vi "U01_TCP_P2PWRITE.vi"() -> ()   [LabVIEW 2015]
doc: "Este VI funciona como un cliente para enviar una cadena"
panel:
  in  "Data in":string="HOLA"
  out "bytes written":i32
  out "connection ID out":refnum<k5>
  out "error out":errorcluster
  in  "IP adress":string="127.0.0.1"
  in  "Port":u16
  in  "timeout ms":i32
  in  "error in (no error)":errorcluster
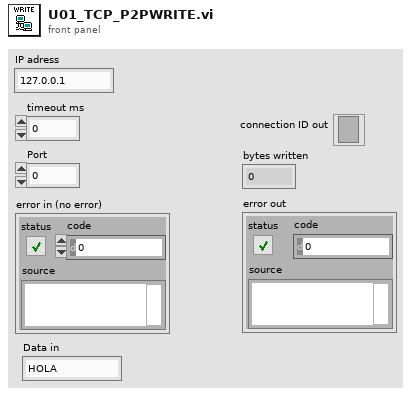
[diagram p1: front panel]
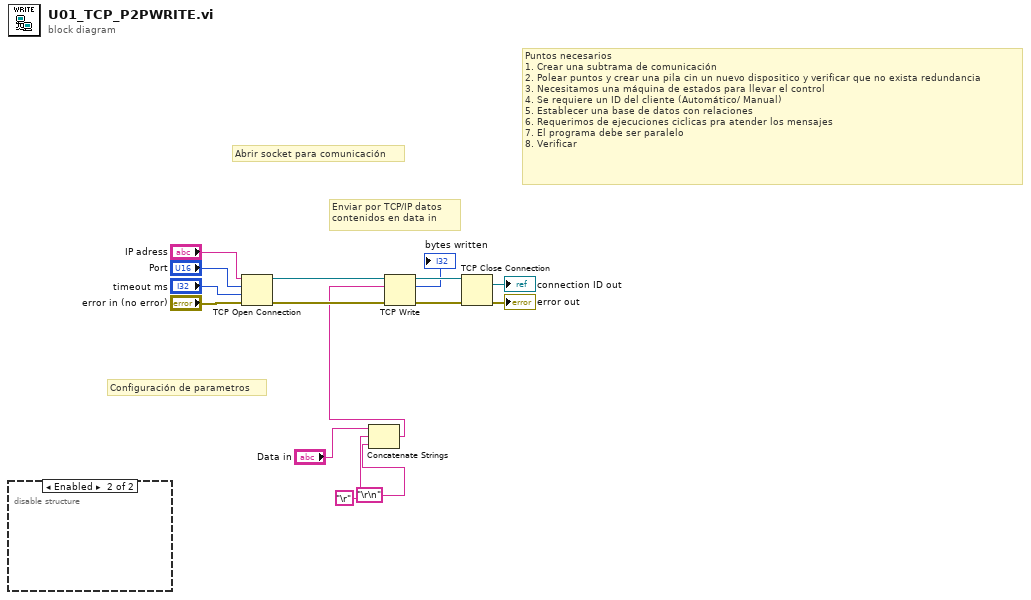
[diagram p0: block diagram]
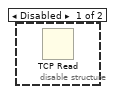
[diagram p2: hidden frame]
diagram:
  # "Abrir socket para comunicación"
  # "Puntos necesarios\n1. Crear una subtrama de comunicación\n2. Polear puntos y crear una pila cin un nuevo dispositico y verificar que no exista redundancia\n3. Necesitamos una máquina de estados para llevar el control\n4. Se requiere un ID del cliente (Automático/ Manual)\n5. Establecer una base de datos con relaciones\n6. Requerimos de ejecuciones ciclicas pra atender los mensajes\n7. El programa debe ser paralelo\n8. Verificar"
  # "Enviar por TCP/IP datos \ncontenidos en data in"
  # "Configuración de parametros"
  n1 = disable-structure shown="Enabled" {
    frame Disabled {
      n2 = TCP Read() -> ()  [unwired: 5 in, 3 out]
    }
    frame Enabled {
    }
  }
  n3 = TCP Open Connection(address="IP adress", remote port or service name="Port", timeout ms (60000)="timeout ms", error in (no error)="error in (no error)") -> (connection ID=w11:refnum<k5>, error out=w10:errorcluster)  [unwired: 1 in]
  n4 = Concatenate Strings("Data in", "\r", "\r\n") -> (w3:string)
  n5 = TCP Write(connection ID=w11, data in=w3, error in (no error)=w10) -> (connection ID out=w8:refnum<k5>, bytes written=→"bytes written":i32, error out=w9:errorcluster)  [unwired: 1 in]
  n6 = TCP Close Connection(connection ID=w8, error in (no error)=w9) -> (connection ID out=→"connection ID out":refnum<k5>, error out=→"error out":errorcluster)  [unwired: 1 in]
